vi "parse solenoids.vi"(0 "Solenoids":T1) -> (1 "Retracted":bool, 2 "Extended":bool)   [LabVIEW 2015]
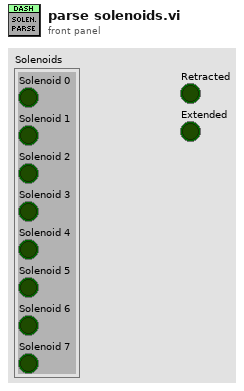
[diagram p1: front panel]
types:
  T1 = cluster{"Solenoid 0":bool, "Solenoid 1":bool, "Solenoid 2":bool, "Solenoid 3":bool, "Solenoid 4":bool, "Solenoid 5":bool, "Solenoid 6":bool, "Solenoid 7":bool}
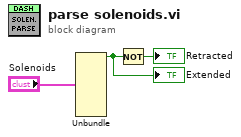
[diagram p0: block diagram]
diagram:
  n1 = Unbundle("Solenoids") -> ("Solenoid 0"=w2:bool)  [unwired: 7 out]
  "Extended" <- w2
  n2 = Not(x=w2) -> (.not. x?=→"Retracted":bool)
